vi "Globals - UI and RT Streams.vi"() -> ()   [LabVIEW 2013]
panel:
  in  "RT Writer Stream":refnum<k21>
  in  "UI Writer Stream":refnum<k21>
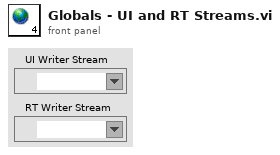
[diagram p1: front panel]
diagram:
